vi "ArchiveDirectory Value Change.vi"(4 "Linux Archive Directory":string caption="Archive Directory", 6 "Windows Archive Directory":path, 7 "Archive Error ref":refnum<vi>, 9 "Linux Paths?":bool, 10 "Event References":T1, 11 "References":T8) -> (0 "error out":errorcluster)   [LabVIEW 2015, in "TDMS datalogger editor node.lvclass"]
uses:
  TDMS datalogger editor node.lvclass
  <vilib>/NI/DCAF/Tag Editor Core/Table API/Table Manager/object ref.ctl
  <vilib>/NI/DCAF/Tag Editor Core/Configuration Editor/Classes/Engine Parent/Engine Parent Editor Node.lvclass
  <vilib>/NI/DCAF/Tag Editor Core/Configuration Editor/Classes/Module editor node/module editor node.lvclass
  <vilib>/NI/DCAF/Tag Editor Core/Table API/Table Manager/references.ctl
  <vilib>/NI/Configuration Framework/Node/StopEvent.ctl
  <vilib>/NI/Configuration Framework/Node/RefreshUIEvent.ctl
  <vilib>/NI/Configuration Framework/Node/CacheState.ctl
  <vilib>/NI/Configuration Framework/Node/NodeChangeEvent.ctl
  <vilib>/NI/Configuration Framework/Node/NodeRef.ctl
  <vilib>/NI/Configuration Framework/Node/NISE_CEF_Node.lvclass
  <vilib>/NI/DCAF/Tag Editor Core/Table API/Available Tag Menu/channel action event.ctl
  <vilib>/NI/DCAF/Tag Editor Core/Table API/Available Tag Menu/dialog output action.ctl
  <vilib>/NI/Tag Bus Module Framework/channel/TBM channel.lvclass
  <vilib>/NI/Tag Bus/tag/tag descriptor.lvclass
  <vilib>/NI/DCAF/Tag Editor Core/Table API/Table Manager/Call Back Ref Type Def.ctl
  <vilib>/NI/AMC/Message Queue.ctl
  <vilib>/NI/AMC/Message.ctl
  <vilib>/NI/Tools/Keyed Array/KeyedArray.ctl
  <vilib>/NI/Configuration Framework/Node/UserEventRef.ctl
  <vilib>/NI/Configuration Framework/Controls/EventCluster.ctl
  TDMS datalogger editor node.lvclass/TDMS datalogger editor node.ctl
  module/configuration/TDMS datalogger configuration.lvclass/TDMS datalogger configuration.ctl
  module/configuration/Write backup directory.vi
  module/configuration/TDMS datalogger configuration.lvclass
  <vilib>/NI/DCAF/Tag Editor Core/Table API/Table Manager/Table Manager.lvclass
  <vilib>/NI/DCAF/Tag Editor Core/Table API/Table Manager.lvlib
  <vilib>/NI/Tools/Keyed Array/Tools_KeyedArray.lvlib
  <vilib>/NI/AMC/AMC.lvlib
  <vilib>/NI/Configuration Framework/NISE_CEF_TreeControl.lvlib
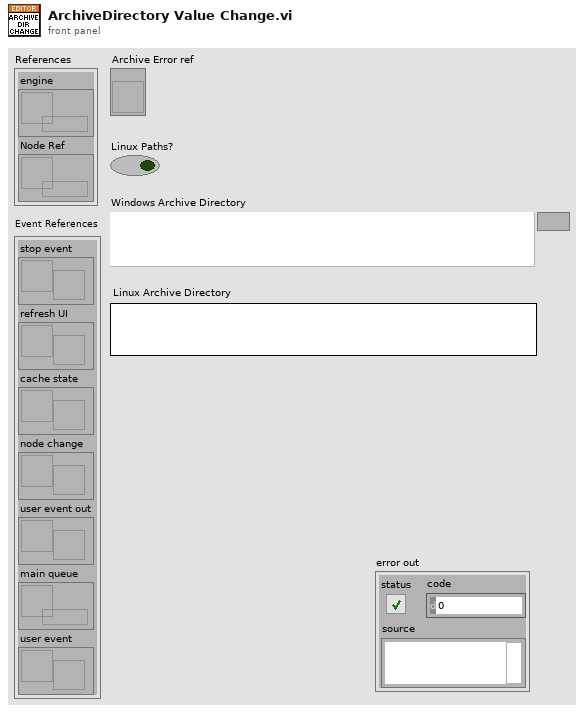
[diagram p1: front panel]
types:
  T1 = typedef "Table Manager.lvlib/Table Manager.lvclass/references.ctl" = cluster{"stop event":T2, "refresh UI":T3, "cache state":T4, "node change":T5, "user event out":refnum<user-event>, "main queue":T6, "user event":T7}
  T2 = typedef "NISE_CEF_Node.lvclass/StopEvent.ctl" = refnum<user-event>
  T3 = typedef "NISE_CEF_Node.lvclass/RefreshUIEvent.ctl" = refnum<user-event>
  T4 = typedef "NISE_CEF_Node.lvclass/CacheState.ctl" = refnum<user-event>
  T5 = typedef "NISE_CEF_Node.lvclass/NodeChangeEvent.ctl" = refnum<user-event>
  T6 = typedef "AMC.lvlib/Message Queue.ctl" = refnum<queue>
  T7 = typedef "NISE_CEF_Node.lvclass/UserEventRef.ctl" = refnum<user-event>
  T8 = typedef "Table Manager.lvlib/Table Manager.lvclass/object ref.ctl" = cluster{"engine":refnum<data-value>, "Node Ref":refnum<data-value>}
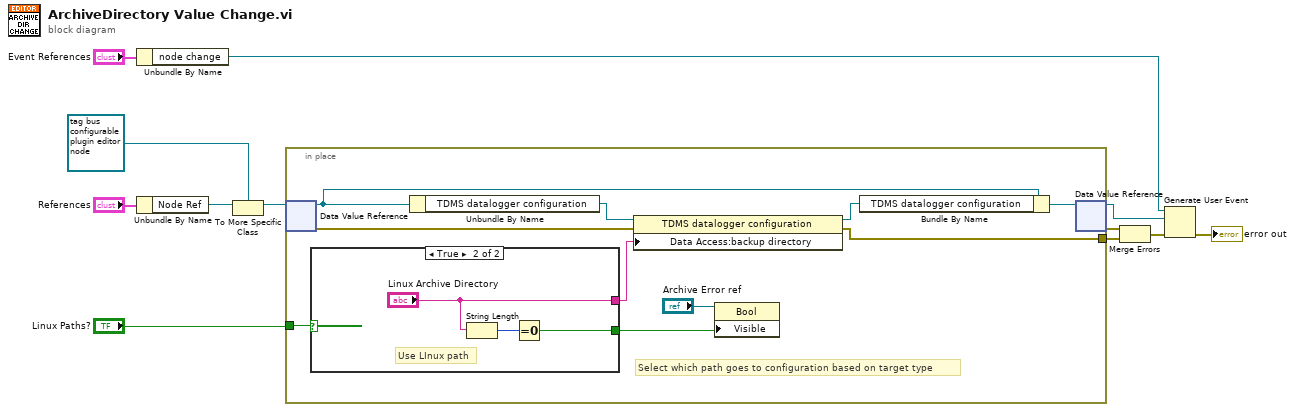
[diagram p0: block diagram]
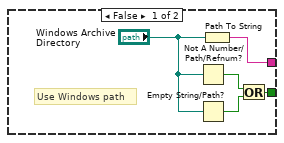
[diagram p2: hidden frame]
diagram:
  n1 = Unbundle By Name("Event References") -> ("node change"=w2:T5)
  n2 = Unbundle By Name("References") -> ("Node Ref"=w11:refnum<data-value>)
  n3 = To More Specific Class(target class=refnum<data-value> refnum ("data value reference"), reference=w11) -> (specific class reference=w8:refnum<data-value>)  [unwired: 1 in, 1 out]
  n4 = in-place {
    in-place-border: [w19] -> w6
    in-place-border: "Linux Paths?" -> [w14]
    # "Select which path goes to configuration based on target type"
    n5 = in-place-dvr #1(w8) -> (w21:refnum<class "TDMS datalogger editor node.lvclass">, w16:errorcluster)
    n6 = case shown="True" w14 {
      tunnel: [w24 w28] -> w20
      tunnel: [w23 "Linux Archive Directory"] -> w15
      frame False {
        # "Use Windows path"
        n7 = Not A Number/Path/Refnum?(number/path/refnum="Windows Archive Directory") -> (NaN/Path/Refnum?=w26:bool)
        n8 = Empty String/Path?(string/path="Windows Archive Directory") -> (empty?=w27:bool)
        n9 = Path To String(path="Windows Archive Directory") -> (string=w23:string)
        n10 = Or(x=w26, y=w27) -> (x .or. y?=w24:bool)
      }
      frame True {
        # "Use LInux path"
        n11 = String Length(string="Linux Archive Directory") -> (length=w29:i32)
        n12 = Equal To 0?(x=w29) -> (x = 0?=w28:bool)
      }
    }
    n13 = Unbundle By Name(w21) -> ("TDMS datalogger configuration"=w17:refnum<class "TDMS datalogger configuration.lvclass">)
    n14 = property class="TDMS datalogger configuration"(reference=w17, error in=w16, "Data Access:backup directory"=w15) -> (reference out=w18:refnum<class "TDMS datalogger configuration.lvclass">, error out=w19:errorcluster)
    n15 = property on="Property Node" class="Bool"(reference="Archive Error ref", "Visible"=w20) -> ()  [unwired: 1 in, 2 out]
    n16 = Bundle By Name(cluster=w21, "TDMS datalogger configuration"=w18) -> (w22:refnum<class "TDMS datalogger editor node.lvclass">)
    n17 = in-place-dvr #1(w22) -> (w1:refnum<data-value>, w5:errorcluster)
  }
  n18 = Merge Errors(w5, w6) -> (w4:errorcluster)
  n19 = Generate User Event(user event=w2, event data cluster=w1, error in=w4) -> (error out=→"error out":errorcluster)  [unwired: 1 in, 1 out]
